vi "Test MQTT-2.3.1-7.vi"(8 "error in (no error)":errorcluster) -> (0 "error out":errorcluster)   [LabVIEW 2013]
uses:
  source/Control Packets/SUBSCRIBE/Topic Subscription -- cluster.ctl
  source/Control Packets/ControlPacket/QualityOfService -- enum.ctl
  source/Client/Client.lvclass
  <vilib>/addons/_JKI Toolkits/Caraya/classes/Assert/Assert Not Equal Value_Variant.vi
  <vilib>/addons/_JKI Toolkits/Caraya/classes/Test/Test.lvclass
  source/Control Packets/ControlPacket/ControlPacket.lvclass
  source/Control Packets/SUBSCRIBE/SUBSCRIBE.lvclass
  source/MQTT_Base/MQTT_Base.lvclass
  <vilib>/addons/_JKI Toolkits/Caraya/classes/Assert/Assert.lvclass
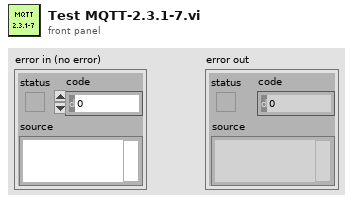
[diagram p1: front panel]
types:
  T1 = typedef "SUBSCRIBE.lvclass/Topic Subscription -- cluster.ctl" = cluster{"Topic Filter":string, "QoS":T2}
  T2 = typedef "ControlPacket.lvclass/QualityOfService -- enum.ctl" = enum16{"0 (At Most Once)", "1 (At Least Once)", "2 (Exactly Once)"}
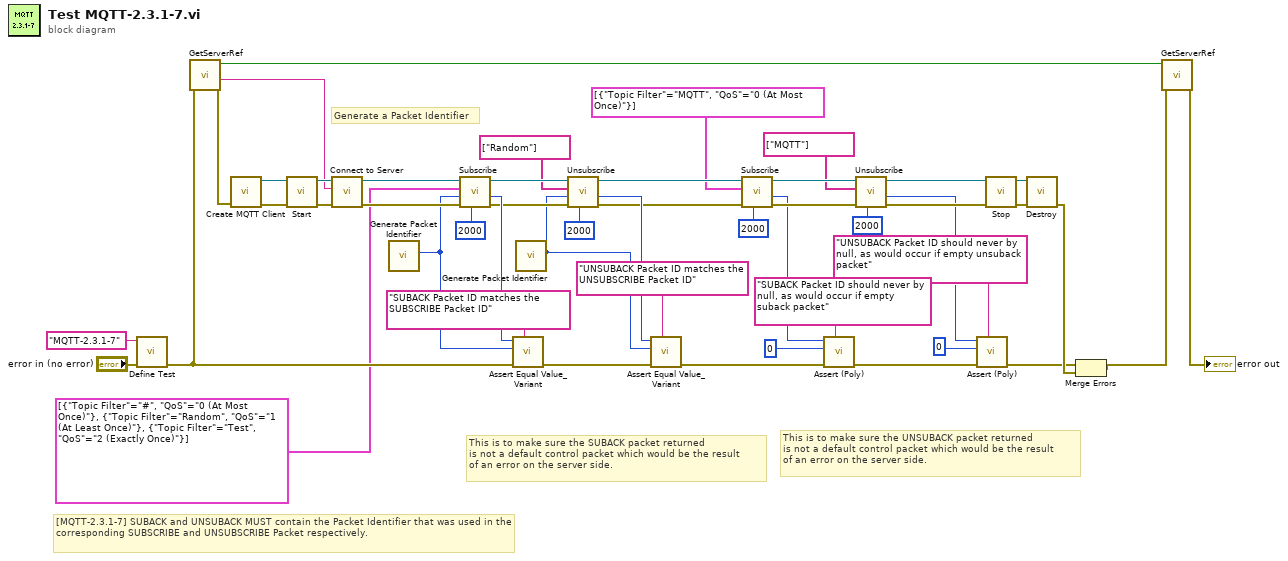
[diagram p0: block diagram]
diagram:
  # "This is to make sure the UNSUBACK packet returned\nis not a default control packet which would be the result\nof an error on the server side."
  # "This is to make sure the SUBACK packet returned\nis not a default control packet which would be the result\nof an error on the server side."
  # "Generate a Packet Identifier"
  # "[MQTT-2.3.1-7] SUBACK and UNSUBACK MUST contain the Packet Identifier that was used in the corresponding SUBSCRIBE and UNSUBSCRIBE Packet respectively."
  n1 = call <vilib>:"Define Test.vi"("error in (no error)"="error in (no error)", "Label (VI Title)"="MQTT-2.3.1-7") -> ("error out"=w33:errorcluster)  [unwired: 9 in]
  n2 = call "GetServerRef.vi"("error in"=w33) -> ("error out"=w46:errorcluster, "Server address"=w28:string, "Created"=w47:bool)  [unwired: 7 in, 1 out]
  n3 = call "Create MQTT Client.vi"("error in (no error)"=w46) -> ("error out"=w35:errorcluster, "Client out"=w36:refnum<class "Client.lvclass">)  [unwired: 9 in]
  n4 = call "Start.vi"("error in (no error)"=w35, "MQTT_Base in"=w36) -> ("error out"=w42:errorcluster, "MQTT_Base out"=w43:refnum<class "Client.lvclass">)  [unwired: 7 in, 1 out]
  n5 = call "Connect to Server.vi"("error in (no error)"=w42, "address (localhost)"=w28, "Client in"=w43) -> ("error out"=w38:errorcluster, "Client out"=w39:refnum<class "Client.lvclass">)  [unwired: 5 in, 2 out]
  n6 = call "Generate Packet Identifier.vi"() -> ("Packet Identifier"=w29:u16)  [unwired: 11 in]
  n7 = call "Subscribe.vi"("timeout (1000 ms)"=2000, "error in (no error)"=w38, "Packet ID (empty: Generate new)"=w29, "Topic Subscriptions"=T1[] [{"Topic Filter"="#", "QoS"=enum."0 (At Most Once)"}, {"Topic Filter"="Random", "QoS"=enum."1 (At Least Once)"}, {"Topic Filter"="Test", "QoS"=enum."2 (Exactly Once)"}], "MQTT_Base in"=w39) -> ("error out"=w26:errorcluster, "SUBACK Packet ID"=w30:u16, "MQTT_Base out"=w27:refnum<class "Client.lvclass">)  [unwired: 3 in, 1 out]
  n8 = call <vilib>:"Assert Equal Value_Variant.vi"("Label"="SUBACK Packet ID matches the SUBSCRIBE Packet ID", "error in (no error)"=w33, "Y"=w29, "X"=w30) -> ("error out"=w23:errorcluster)  [unwired: 7 in]
  n9 = call "Generate Packet Identifier.vi"() -> ("Packet Identifier"=w20:u16)  [unwired: 11 in]
  n10 = call "Unsubscribe.vi"("timeout (1000 ms)"=2000, "error in (no error)"=w26, "Packet ID (empty: Generate new)"=w20, "Topics"=string[] ["Random"], "MQTT_Base in"=w27) -> ("error out"=w18:errorcluster, "UNSUBACK Packet ID"=w22:u16, "MQTT_Base out"=w19:refnum<class "Client.lvclass">)  [unwired: 4 in]
  n11 = call <vilib>:"Assert Equal Value_Variant.vi"("Label"="UNSUBACK Packet ID matches the UNSUBSCRIBE Packet ID", "error in (no error)"=w23, "Y"=w20, "X"=w22) -> ("error out"=w9:errorcluster)  [unwired: 7 in]
  n12 = call "Subscribe.vi"("timeout (1000 ms)"=2000, "error in (no error)"=w18, "Topic Subscriptions"=T1[] [{"Topic Filter"="MQTT", "QoS"=enum."0 (At Most Once)"}], "MQTT_Base in"=w19) -> ("error out"=w14:errorcluster, "SUBACK Packet ID"=w8:u16, "MQTT_Base out"=w15:refnum<class "Client.lvclass">)  [unwired: 4 in, 1 out]
  n13 = call-poly <vilib>:"Assert (Poly).vi"("Label"="SUBACK Packet ID should never by null, as would occur if empty suback packet", "error in (no error)"=w9, "Y"=u16 0 ("SUBACK Packet ID"), "X"=w8) -> ("error out"=w5:errorcluster)  [unwired: 7 in]
  n14 = call "Unsubscribe.vi"("timeout (1000 ms)"=2000, "error in (no error)"=w14, "Topics"=string[] ["MQTT"], "MQTT_Base in"=w15) -> ("error out"=w13:errorcluster, "UNSUBACK Packet ID"=w2:u16, "MQTT_Base out"=w12:refnum<class "Client.lvclass">)  [unwired: 5 in]
  n15 = call-poly <vilib>:"Assert (Poly).vi"("Label"="UNSUBACK Packet ID should never by null, as would occur if empty unsuback packet", "error in (no error)"=w5, "Y"=u16 0 ("SUBACK Packet ID"), "X"=w2) -> ("error out"=w4:errorcluster)  [unwired: 7 in]
  n16 = call "Stop.vi"("error in (no error)"=w13, "MQTT_Base in"=w12) -> ("error out"=w40:errorcluster, "MQTT_Base out"=w41:refnum<class "Client.lvclass">)  [unwired: 7 in, 1 out]
  n17 = call-dynamic "Destroy.vi"("error in (no error)"=w40, "MQTT_Base in"=w41) -> ("error out"=w31:errorcluster)  [unwired: 8 in, 1 out]
  n18 = Merge Errors(w4, w31) -> (w34:errorcluster)
  n19 = call "GetServerRef.vi"("error in"=w34, "Destroy (F)"=w47) -> ("error out"=→"error out":errorcluster)  [unwired: 6 in, 3 out]
